vi "DB Tools Get Parameter Value.vi"   [LabVIEW 2017, in "NI_Database_API.lvlib"]
doc: "Retrieves the value of the parameter specified by the <B>parameter index</B> input in the command or command-recordset. The <B>parameter index</B> can be either the zero-indexed position of the parameter in the command or the name of the parameter. Wire data to the <B>type</B> input to determine the polymorphic instance to use or manually select the instance."
uses:
  <vilib>/addons/database/NI_Database_API.lvlib
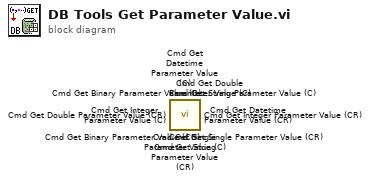
[diagram p0: block diagram]
diagram:
  n1 = call <vilib>:"Cmd Get Single Parameter Value (C).vi"() -> ()  [unwired: 7 in, 3 out]
  n2 = call <vilib>:"Cmd Get Double Parameter Value (C).vi"() -> ()  [unwired: 7 in, 3 out]
  n3 = call <vilib>:"Cmd Get Integer Parameter Value (C).vi"() -> ()  [unwired: 7 in, 3 out]
  n4 = call <vilib>:"Cmd Get Datetime Parameter Value (CR).vi"() -> ()  [unwired: 7 in, 3 out]
  n5 = call <vilib>:"Cmd Get Binary Parameter Value (C).vi"() -> ()  [unwired: 7 in, 3 out]
  n6 = call <vilib>:"Cmd Get Datetime Parameter Value (C).vi"() -> ()  [unwired: 7 in, 3 out]
  n7 = call <vilib>:"Cmd Get Single Parameter Value (CR).vi"() -> ()  [unwired: 7 in, 3 out]
  n8 = call <vilib>:"Cmd Get String Parameter Value (CR).vi"() -> ()  [unwired: 7 in, 3 out]
  n9 = call <vilib>:"Cmd Get Double Parameter Value (CR).vi"() -> ()  [unwired: 7 in, 3 out]
  n10 = call <vilib>:"Cmd Get Integer Parameter Value (CR).vi"() -> ()  [unwired: 7 in, 3 out]
  n11 = call <vilib>:"Cmd Get Binary Parameter Value (CR).vi"() -> ()  [unwired: 7 in, 3 out]
  n12 = call <vilib>:"Cmd Get String Parameter Value (C).vi"() -> ()  [unwired: 7 in, 3 out]
